vi "V3SVTest(copy).vi"() -> ()   [LabVIEW 2011]
uses:
  <instrlib>/Voltech PM1000+/Public/Configure/Configure Measurements (Normal).vi
  <vilib>/Utility/file.llb/Write To Spreadsheet File (string).vi
  <instrlib>/Voltech PM1000+/Voltech PM1000+.lvlib
panel:
  in  "Minutes per test":dbl
  in  "FOLDER NAME":string
  in  "HOW MANY TEST":i32
  in  "Name of File":string
  in  "VISA resource name 2":refnum<visa-resource-name>
  out "Current Data Point":i32
  in  "stop":bool
  out "Watts":dbl[](graph)
  in  "Normal Measurements":i32[](listbox)=[0, 1, 2, 3, 4, 5, 6]
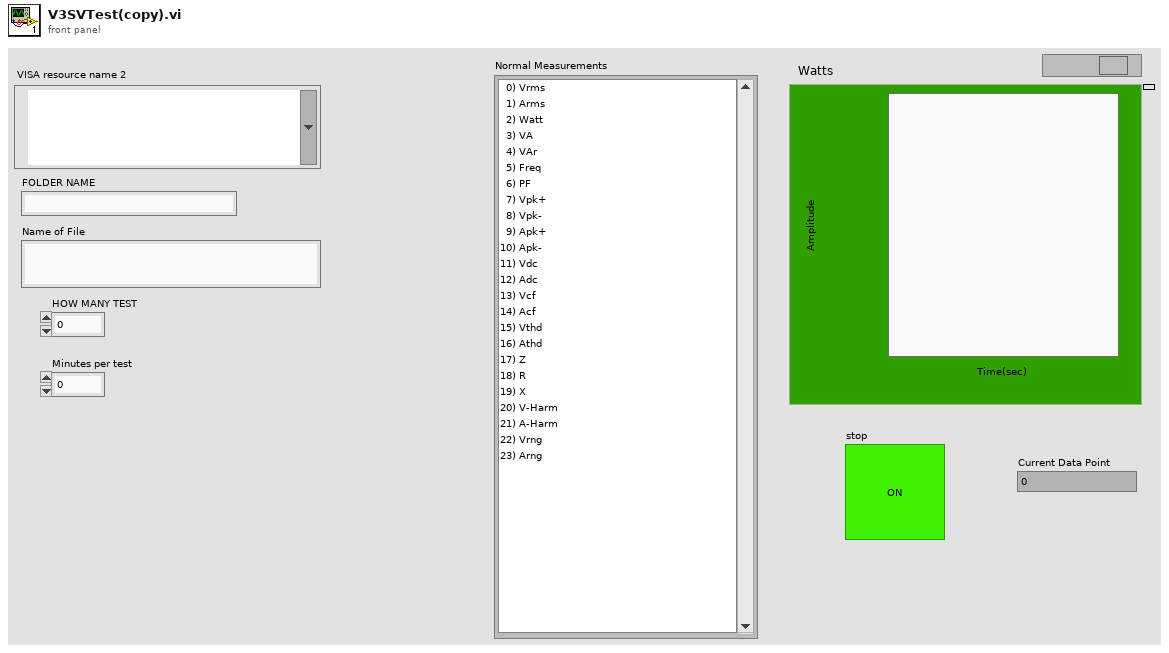
[diagram p1: front panel]
types:
  T1 = enum16{"open", "replace", "create", "open or create", "replace or create", "replace or create with confirmation"}
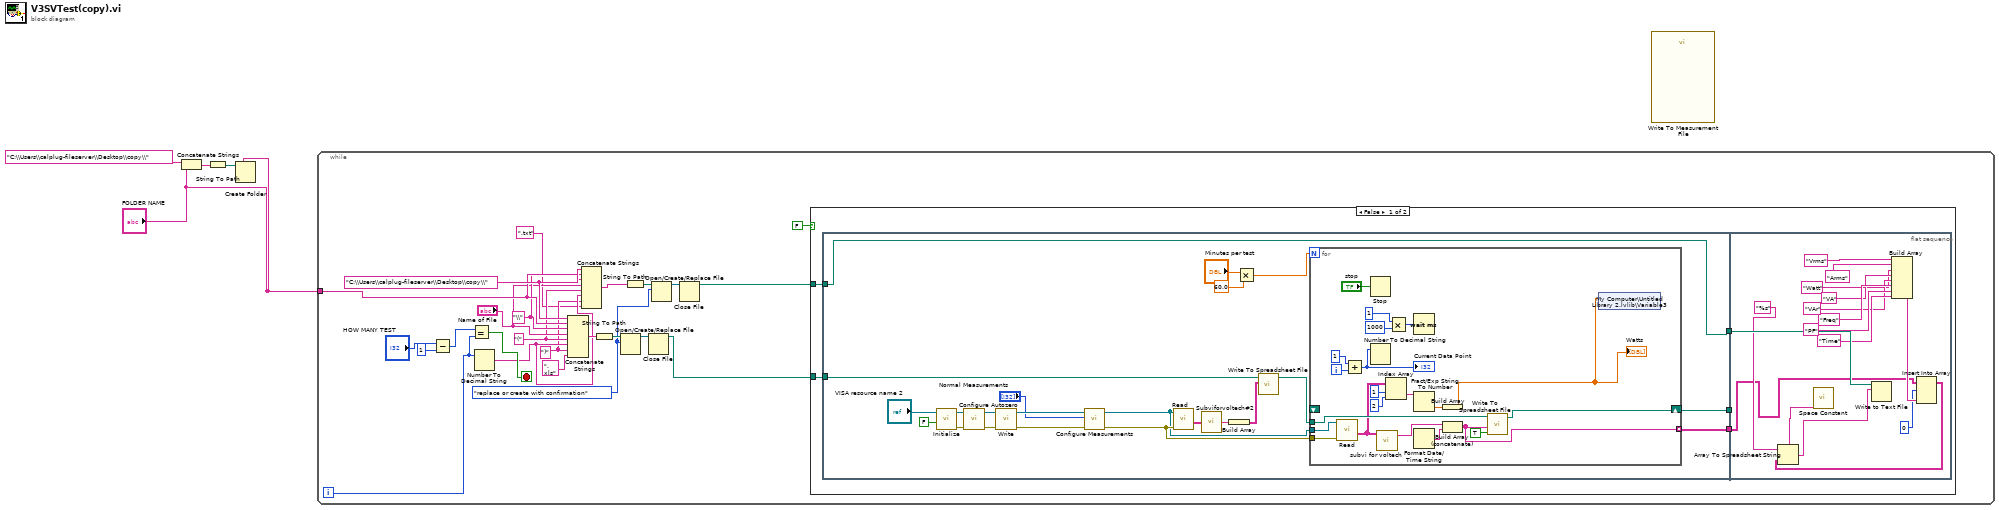
[diagram p0: block diagram]
diagram:
  n1 = Concatenate Strings("C:\\Users\\calplug-fileserver\\Desktop\\copy\\" ("string"), "FOLDER NAME") -> (w4:string)
  n2 = String To Path(string=w4) -> (path=w3:path)
  n3 = Create Folder(prompt (Create Folder)="FOLDER NAME", path (use dialog)=w3) -> ()  [unwired: 1 in, 3 out]
  n4 = while {
    tunnel: "FOLDER NAME" -> [w16]
    i -> [w21]
    stop <- w22 stop-if-true
    w15 = "\\" ("string")
    w11 = ")" ("string")
    w13 = "(" ("string")
    w6 = T1."replace or create with confirmation" ("operation (0:open)")
    w17 = "C:\\Users\\calplug-fileserver\\Desktop\\copy\\" ("string")
    n5 = Subtract(x="HOW MANY TEST", y=1) -> (x-y=w18:i32)
    n6 = Equal?(x=w18, y=w21) -> (x = y?=w22:bool)
    n7 = Number To Decimal String(number=w21) -> (decimal integer string=w12:string)  [unwired: 1 in]
    n8 = Concatenate Strings(w17, w16, w15, "Name of File", w13, w12, w11, ".xls" ("string")) -> (w26:string)
    n9 = Concatenate Strings(w17, w16, w15, "Name of File", w13, w12, w11, ".txt") -> (w7:string)
    n10 = String To Path(string=w26) -> (path=w27:path)
    n11 = Open/Create/Replace File(file path (use dialog)=w27, operation (0:open)=w6) -> (refnum out=w25:refnum<file>)  [unwired: 4 in, 2 out]
    n12 = String To Path(string=w7) -> (path=w9:path)
    n13 = Close File(refnum=w25) -> (path=w23:path)  [unwired: 1 in, 1 out]
    n14 = Open/Create/Replace File(file path (use dialog)=w9, operation (0:open)=w6) -> (refnum out=w8:refnum<file>)  [unwired: 4 in, 2 out]
    n15 = Close File(refnum=w8) -> (path=w5:path)  [unwired: 1 in, 1 out]
    n16 = case shown="False" FALSE {
      tunnel: w23 -> [w33 _]
      tunnel: w5 -> [w31 _]
      frame False {
        n17 = flat-sequence {
          tunnel: w33 -> [w45]
          tunnel: [w51] -> w32
          tunnel: w31 -> [w35]
          tunnel: [w35] -> w30
          tunnel: [w34] -> w29
          tunnel: w32 -> [_]
          tunnel: w30 -> [w92]
          tunnel: w29 -> [w79]
          frame #0 {
            n18 = call <instrlib>:"Initialize.vi"("Reset (True)"=FALSE, "VISA resource name"="VISA resource name 2") -> ("error out"=w53:errorcluster, "VISA resource name out"=w54:refnum<visa-resource-name>)  [unwired: 8 in]
            n19 = call <instrlib>:"Configure Autozero.vi"("error in (no error)"=w53, "VISA resource name"=w54) -> ("error out"=w49:errorcluster, "VISA resource name out"=w50:refnum<visa-resource-name>)  [unwired: 8 in]
            n20 = call <instrlib>:"Write.vi"("error in (no error)"=w49, "VISA resource name"=w50) -> ("error out"=w47:errorcluster, "VISA resource name out"=w48:refnum<visa-resource-name>)  [unwired: 8 in]
            n21 = call-poly <instrlib>:"Configure Measurements.vi"("error in (no error)"=w47, "Normal Measurements"="Normal Measurements", "VISA resource name"=w48) -> ("error out"=w41:errorcluster, "VISA resource name out"=w40:refnum<visa-resource-name>)  [unwired: 7 in]
            n22 = call <instrlib>:"Read.vi"("error in (no error)"=w41, "VISA resource name"=w40) -> ("Measurement Results"=w42:string[][])  [unwired: 7 in, 2 out]
            n23 = call "Subviforvoltech#2.vi"("Measurement Results 2"=w42) -> ("Array"=w46:string[])
            n24 = Build Array(w46) -> (w36:string[][])
            n25 = Multiply(x="Minutes per test", y=60.0) -> (x*y=w39:dbl)
            n26 = call-poly <vilib>:"Write To Spreadsheet File.vi"("2D data"=w36, "file path (dialog if empty)"=w45) -> ("new file path (Not A Path if cancelled)"=w44:path)  [unwired: 6 in]
            n27 = for {
              N: w39 -> [_]
              tunnel: w44 -> [w71]
              shift-right: [w69] -> w51
              shift-left: _ -> [_]
              tunnel: w40 -> [w68]
              tunnel: w41 -> [w67]
              tunnel: [w56] -> w34 mode=indexing
              i -> [w73]
              n28 = call <instrlib>:"Read.vi"("error in (no error)"=w67, "VISA resource name"=w68) -> ("Measurement Results"=w58:string[][])  [unwired: 7 in, 2 out]
              n29 = Add(x=1, y=w73) -> (x+y=w74:i32)
              "Current Data Point" <- w74
              n30 = Stop(stop? (T)="stop") -> ()
              n31 = Number To Decimal String(number=w74) -> ()  [unwired: 1 in, 1 out]
              n32 = call "subvi for voltech.vi"("Measurement Results 2"=w58) -> ("Array"=w59:string[])  [unwired: 6 in]
              n33 = Index Array(array=w58, index (row)=1, index (col)=2 ("disabled index (col)")) -> (element=w57:string)
              n34 = Multiply(x=u32 1 ("Interval of Data Collection (sec)"), y=u32 1000) -> (x*y=w75:u32)
              n35 = Wait (ms)(milliseconds to wait=w75) -> ()  [unwired: 1 out]
              n36 = Fract/Exp String To Number(string=w57) -> (number=w61:dbl)  [unwired: 3 in, 1 out]
              n37 = Format Date/Time String() -> (date/time string=w65:string)  [unwired: 3 in]
              n38 = Build Array(w61) -> (w60:dbl[])
              "Watts" <- w60
              n39 = Build Array (concatenate)(w59, w65) -> (w56:string[])
              n40 = call-poly <vilib>:"Write To Spreadsheet File.vi"("append to file? (new file:F)"=TRUE, "1D data"=w56, "file path (dialog if empty)"=w71) -> ("new file path (Not A Path if cancelled)"=w69:path)  [unwired: 5 in]
              n41 = shared-variable "My Computer\\Untitled Library 2.lvlib\\Variable3"(w60) -> ()  [unwired: 1 in, 1 out]
            }
          }
          frame #1 {
            n42 = call <vilib>:"Space Constant.vi"() -> ("String"=w89:string)
            n43 = Build Array("Vrms", "Arms", "Watt", "VA", "VAr", "Freq", "PF", "Time") -> (w80:string[])
            n44 = Insert Into Array(array=w79, index (row)=0, new element=w80) -> (w78:string[][])  [unwired: 1 in]
            n45 = Array To Spreadsheet String(delimiter (Tab)=w89, array=w78, 3:"%s") -> (spreadsheet string=w91:string)
            n46 = Write to Text File(file (use dialog)=w92, text=w91) -> ()  [unwired: 2 in, 3 out]
          }
        }
      }
      frame True {
      }
    }
  }
  n47 = call "Write To Measurement File"() -> ()  [unwired: 17 in, 3 out]
